vi "Test Permitions.vi"() -> ()   [LabVIEW 2016]
panel:
  out "standard output 2":string
  out "standard output":string
  out "standard error":string
  in  "# Points":i32
  in  "File Path Control":path=path "C:/Data/test.tdms"
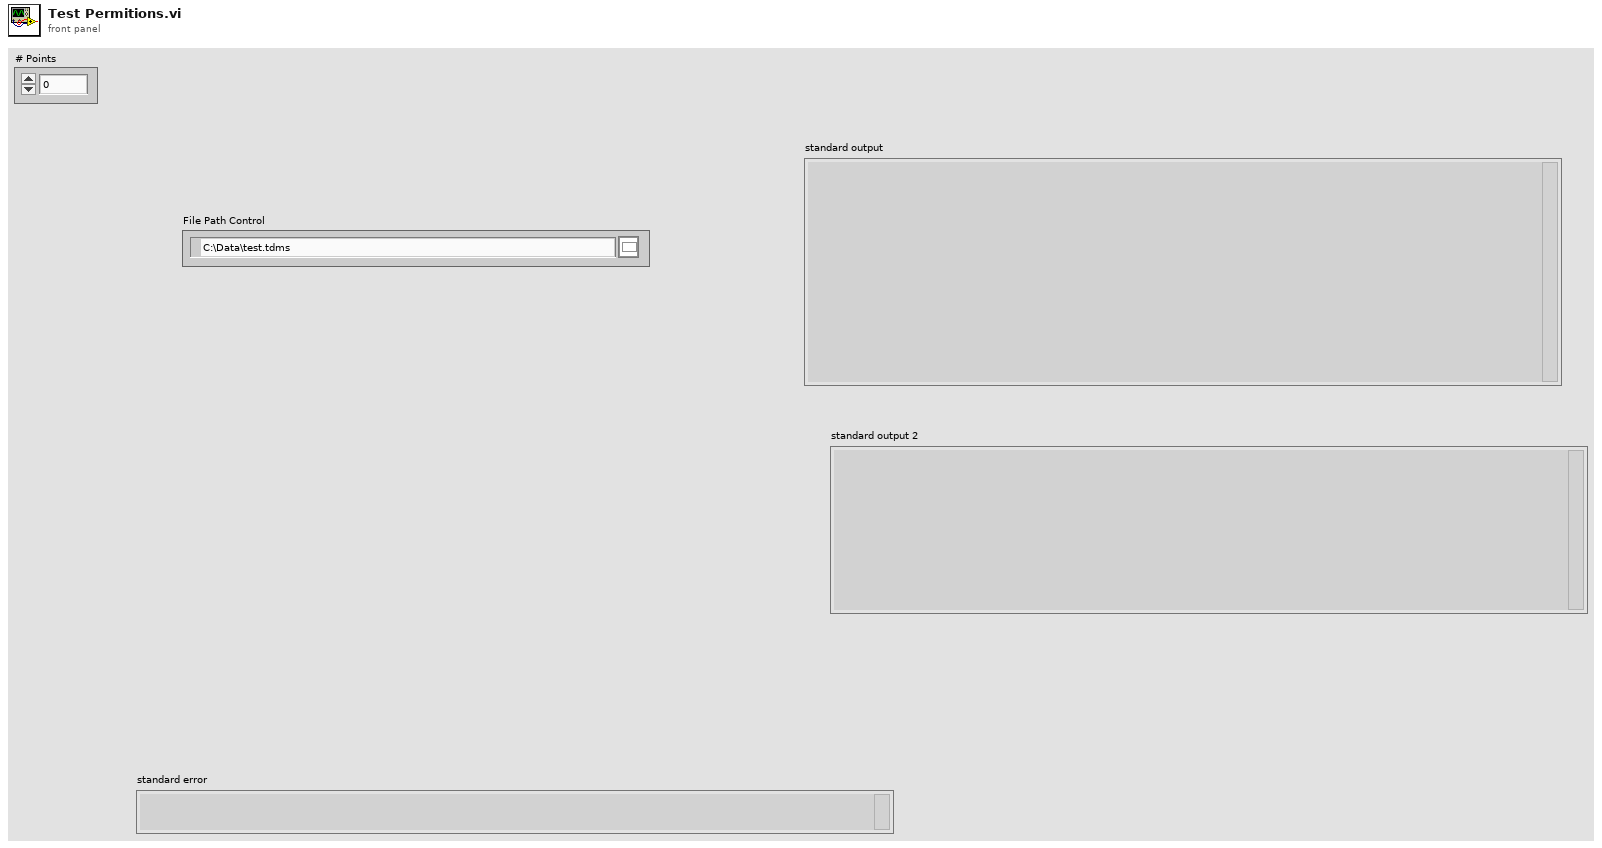
[diagram p1: front panel]
types:
  T1 = enum16{"open", "open or create", "create or replace", "create", "open (read-only)"}
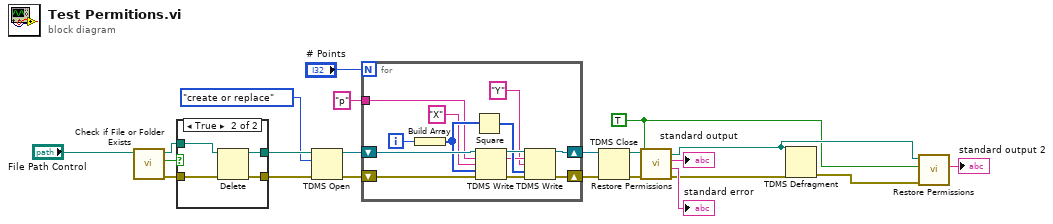
[diagram p0: block diagram]
diagram:
  w2 = TRUE ("View only")
  n1 = call <vilib>:"Check if File or Folder Exists.vi"("path"="File Path Control") -> ("error out"=w20:errorcluster, "file or folder exists?"=w22:bool, "dup path"=w21:path)  [unwired: 8 in]
  n2 = case shown="True" w22 {
    tunnel: w21 -> [w24 w28]
    tunnel: w20 -> [w23 w27]
    tunnel: [w24 w26] -> w18
    tunnel: [w23 w25] -> w17
    frame False {
    }
    frame True {
      n3 = Delete(path (use dialog)=w28, error in=w27) -> (deleted path=w26:path, error out=w25:errorcluster)  [unwired: 3 in, 1 out]
    }
  }
  n4 = TDMS Open(8:w17, 10:T1."create or replace" ("operation (0:open)"), 11:w18) -> (0:w13:errorcluster, 3:w14:refnum<k34>)  [unwired: 4 in]
  n5 = for {
    N: "# Points" -> [_]
    tunnel: "p" ("group name in (Untitled)") -> [w34]
    shift-right: [w29] -> w10
    shift-left: w14 -> [w41]
    shift-right: [w30] -> w11
    shift-left: w13 -> [w38]
    i -> [w37]
    n6 = Build Array(w37) -> (w36:i32[])
    n7 = Square(x=w36) -> (x^2=w35:i32[])
    n8 = TDMS Write(0:w41, 5:w34, 7:"X" ("group name in (Untitled)"), 9:w36, 11:w38) -> (4:w40:refnum<k34>, 6:w33:string, 15:w39:errorcluster)  [unwired: 1 in, 1 out]
    n9 = TDMS Write(0:w40, 5:w33, 7:"Y" ("group name in (Untitled)"), 9:w35, 11:w39) -> (4:w29:refnum<k34>, 15:w30:errorcluster)  [unwired: 1 in, 2 out]
  }
  n10 = TDMS Close(8:w11, 11:w10) -> (0:w9:errorcluster, 3:w8:path)
  n11 = call "Restore Permissions.vi"("Error In"=w9, "View only"=w2, "File Path"=w8) -> ("Error Out"=w5:errorcluster, "standard error"=→"standard error":string, "standard output"=→"standard output":string, "Duplicate File Path"=w3:path)  [unwired: 5 in]
  n12 = TDMS Defragment(4:w5, 7:w3) -> (0:w4:errorcluster)
  n13 = call "Restore Permissions.vi"("Error In"=w4, "View only"=w2, "File Path"=w3) -> ("standard output"=→"standard output 2":string)  [unwired: 5 in, 3 out]
